vi "table_get_inline_subtable_item.vi"(8 "error in (no error)":errorcluster, 9 "subkeys":string[](array[string]), 11 "Item in":refnum<class "Item.lvclass">) -> (0 "error out":errorcluster, 1 "Item":refnum<class "Item.lvclass">, 2 "contains_item":bool)   [LabVIEW 2020, in "toml.lvclass"]
uses:
  toml.lvclass
  Item/Item.lvclass
  toml.lvclass/toml.ctl
  InlineTable/InlineTable.lvclass
  a6521568-7b9b-4f3a-a21f-e992a05a1e4d.vi
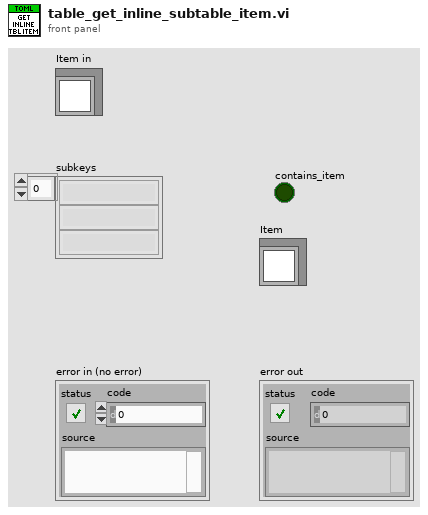
[diagram p1: front panel]
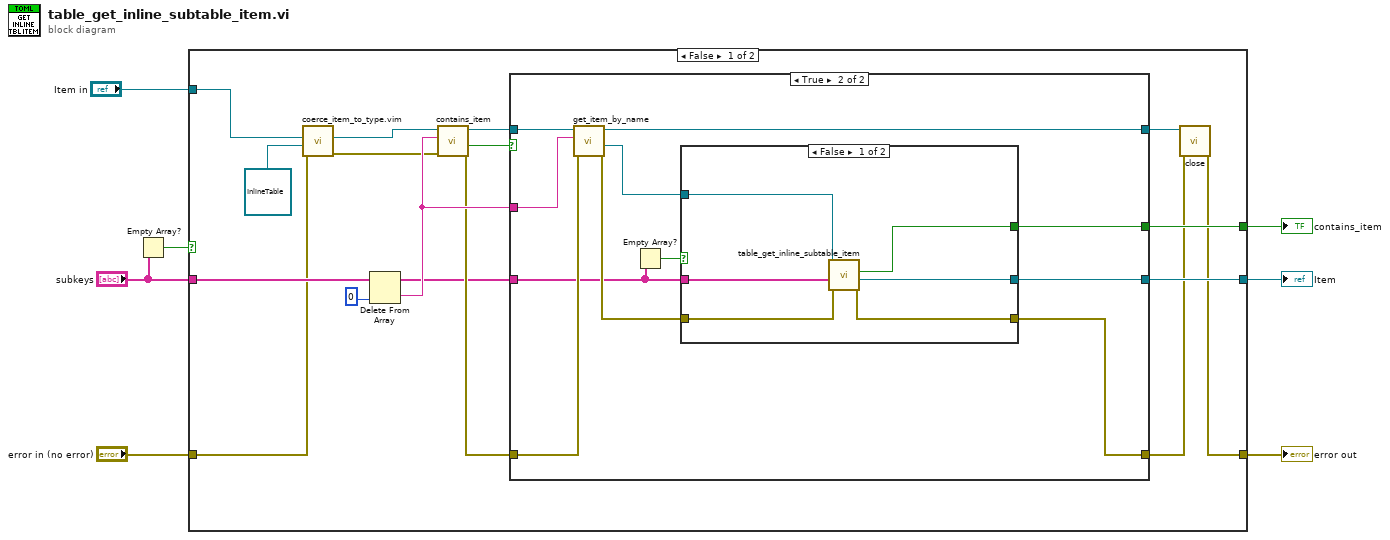
[diagram p0: block diagram]
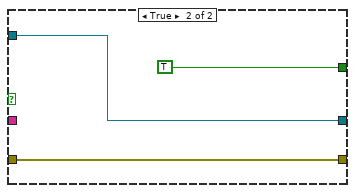
[diagram p3: hidden frame]
diagram:
  n1 = Empty Array?(array="subkeys") -> (empty?=w1:bool)
  n2 = case shown="False" w1 {
    tunnel: "error in (no error)" -> [w8 w47]
    tunnel: "Item in" -> [w11 w48]
    tunnel: [w20 w48] -> w5
    tunnel: [w13 w47] -> w4
    tunnel: [w17 _] -> w3
    tunnel: "subkeys" -> [w16 _]
    frame False {
      n3 = call "coerce_item_to_type.vim"("error in (no error)"=w8, "default (\"\")"=refnum<class "InlineTable.lvclass"> refnum ("Table out"), "Item in"=w11) -> ("error out"=w9:errorcluster, "string_value"=w10:refnum<class "InlineTable.lvclass">)  [unwired: 7 in]
      n4 = Delete From Array(array=w16, index=0) -> (deleted portion=w24:string, array with subset deleted=w19:string[])  [unwired: 1 in]
      n5 = call "contains_item.vi"("error in (no error)"=w9, "key_name"=w24, "Table in"=w10) -> ("error out"=w22:errorcluster, "contains_item"=w18:bool, "Table out"=w21:refnum<class "InlineTable.lvclass">)  [unwired: 6 in]
      n6 = case shown="True" w18 {
        tunnel: w24 -> [_ w37]
        tunnel: w22 -> [w26 w36]
        tunnel: w21 -> [w25 w35]
        tunnel: [_ w33] -> w20
        tunnel: [w26 w28] -> w14
        tunnel: w19 -> [_ w30]
        tunnel: [_ w29] -> w17
        tunnel: [w25 w27] -> w15
        frame False {
        }
        frame True {
          n7 = call "get_item_by_name.vi"("error in (no error)"=w36, "key_name"=w37, "Table in"=w35) -> ("error out"=w31:errorcluster, "Item"=w32:refnum<class "Item.lvclass">, "Table out"=w27:refnum<class "InlineTable.lvclass">)  [unwired: 6 in]
          n8 = Empty Array?(array=w30) -> (empty?=w34:bool)
          n9 = case shown="False" w34 {
            tunnel: [w39 w46] -> w33
            tunnel: w32 -> [w43 w46]
            tunnel: w31 -> [w41 w45]
            tunnel: [w40 w45] -> w28
            tunnel: w30 -> [w42 _]
            tunnel: [w38 TRUE ("contains_item")] -> w29
            frame False {
              n10 = call "table_get_inline_subtable_item.vi"("error in (no error)"=w41, "subkeys"=w42, "Item in"=w43) -> ("error out"=w40:errorcluster, "Item"=w39:refnum<class "Item.lvclass">, "contains_item"=w38:bool)  [unwired: 6 in]
            }
            frame True {
            }
          }
        }
      }
      n11 = call "close.vi"("error in (no error)"=w14, "Table in"=w15) -> ("error out"=w13:errorcluster)  [unwired: 9 in]
    }
    frame True {
    }
  }
  "contains_item" <- w3
  "Item" <- w5
  "error out" <- w4
